vi "mdps daq tmp.vi"(8 "steering":dbl(knob) min=-0.45 max=0.45 step=0.005 scale=-0.45..0.45, 11 "auto":bool) -> ()   [LabVIEW 2015]
uses:
  <vilib>/DAQmx/write.llb/DAQmx Write (Analog 1D DBL NChan 1Samp).vi
  <vilib>/DAQmx/miscellaneous.llb/DAQmx Fill In Error Info.vi
  <vilib>/DAQmx/create/channels.llb/DAQmx Create Channel (AO-Voltage-Basic).vi
panel:
  out "error out":errorcluster
  out "count":i32
  out "AO":refnum<k21>
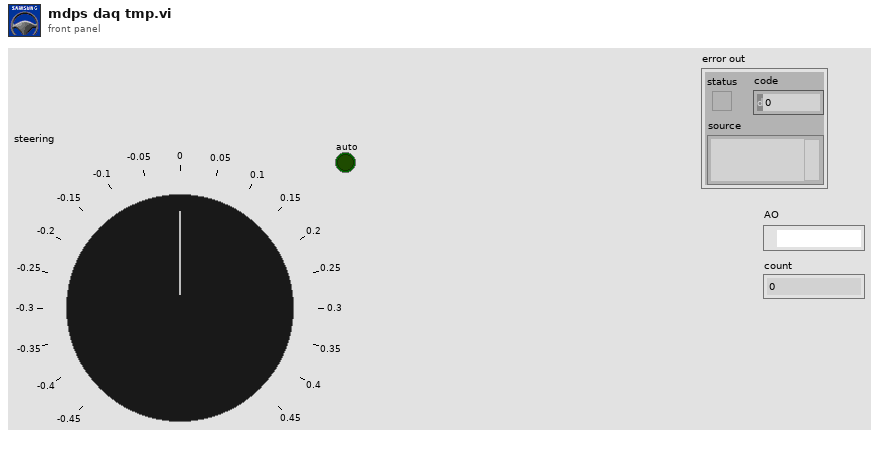
[diagram p1: front panel]
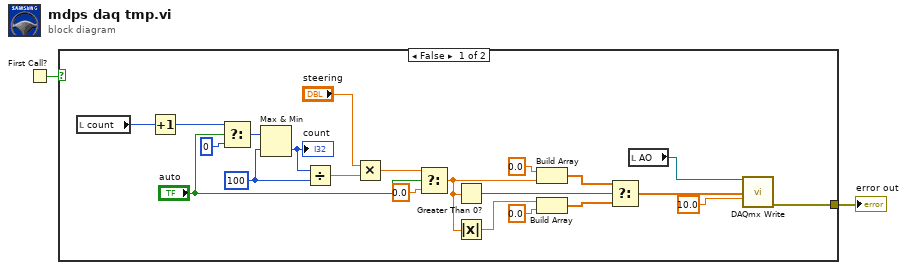
[diagram p0: block diagram]
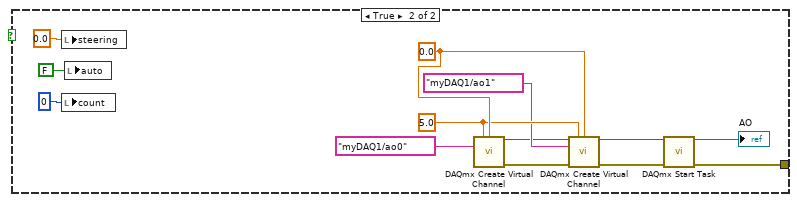
[diagram p2: hidden frame]
diagram:
  n1 = First Call?() -> (First Call?: T/F=w2:bool)
  n2 = case shown="False" w2 {
    tunnel: [w3 w25] -> w1
    frame False {
      w12 = 100 ("y")
      n3 = local read "count"() -> (w13:i32)
      n4 = Increment(x=w13) -> (x+1=w7:i32)
      n5 = Select(t=w7, s="auto", f=0) -> (s? t:f=w6:i32)
      n6 = Max & Min(x=w6, y=w12) -> (min(x,y)=w8:i32)  [unwired: 1 out]
      "count" <- w8
      n7 = Divide(x=w8, y=w12) -> (x/y=w11:dbl)
      n8 = Multiply(x="steering", y=w11) -> (x*y=w9:dbl)
      n9 = Select(t=w9, s="auto", f=0.0) -> (s? t:f=w15:dbl)
      n10 = Greater Than 0?(x=w15) -> (x > 0?=w23:bool)
      n11 = Absolute Value(x=w15) -> (abs(x)=w20:dbl)
      n12 = Build Array(0.0 ("element"), w15) -> (w21:dbl[])
      n13 = Build Array(w20, 0.0 ("element")) -> (w19:dbl[])
      n14 = Select(t=w21, s=w23, f=w19) -> (s? t:f=w17:dbl[])
      n15 = local read "AO"() -> (w14:refnum<k21>)
      n16 = call-poly <vilib>:"DAQmx Write.vi"("task/channels in"=w14, "data"=w17, "timeout"=10.0) -> ("error out"=w3:errorcluster)  [unwired: 10 in, 2 out]
    }
    frame True {
      w32 = 0.0 ("minimum value")
      w31 = 5.0 ("maximum value")
      n17 = local write "steering"(0.0 ("steering")) -> ()
      n18 = local write "count"(0 ("count")) -> ()
      n19 = local write "auto"(FALSE ("auto")) -> ()
      n20 = call-poly <vilib>:"DAQmx Create Virtual Channel.vi"("maximum value"=w31, "minimum value"=w32, "physical channels"=tag "myDAQ1/ao0") -> ("task out"=w29:refnum<k21>, "error out"=w27:errorcluster)  [unwired: 11 in]
      n21 = call-poly <vilib>:"DAQmx Create Virtual Channel.vi"("task in"=w29, "maximum value"=w31, "minimum value"=w32, "physical channels"=tag "myDAQ1/ao1", "error in"=w27) -> ("task out"=w33:refnum<k21>, "error out"=w26:errorcluster)  [unwired: 9 in]
      n22 = call <vilib>:"DAQmx Start Task.vi"("task/channels in"=w33, "error in"=w26) -> ("task out"=→"AO":refnum<k21>, "error out"=w25:errorcluster)  [unwired: 12 in]
    }
  }
  "error out" <- w1
